vi "PicoScope_Ini.vi"() -> (0 "error out":errorcluster, 1 "Max Adc value":i16, 2 "PicoScope Type":string, 3 "handle":i16, 4 "Serial":string, 5 "Device Info":T1)   [LabVIEW 2018]
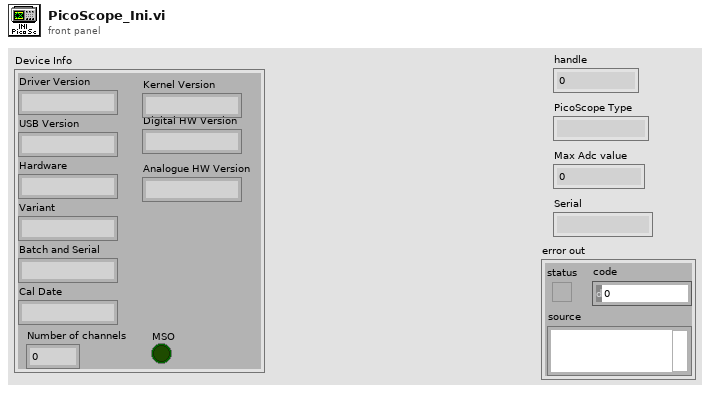
[diagram p1: front panel]
types:
  T1 = cluster{"Driver Version":string, "USB Version":string, "Hardware":string, "Variant":string, "Batch and Serial":string, "Cal Date":string, "Kernel Version":string, "Digital HW Version":string, "Analogue HW Version":string, "MSO":bool, "Number of channels":i16}
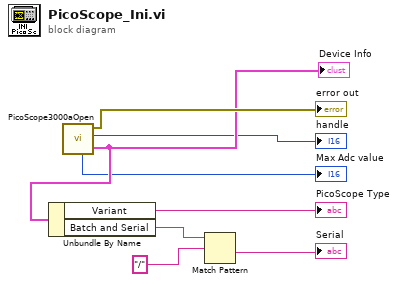
[diagram p0: block diagram]
diagram:
  n1 = call "PicoScope3000aOpen.vi"() -> ("handle"=→"handle":i16, "error out"=→"error out":errorcluster, "Max ADC value"=→"Max Adc value":i16, "Device Info"=w3:T1)  [unwired: 6 in, 2 out]
  "Device Info" <- w3
  n2 = Unbundle By Name(w3) -> ("Variant"=→"PicoScope Type":string, "Batch and Serial"=w7:string)
  n3 = Match Pattern(string=w7, regular expression="/") -> (after substring=→"Serial":string)  [unwired: 1 in, 3 out]
